vi "Read Sudoku String.vi"(8 "error in (no error)":errorcluster, 11 "Sudoku Class in":refnum<class "Sudoku Class.lvclass">) -> (0 "error out":errorcluster, 2 "Sudoku String":T1, 3 "Sudoku Class out":refnum<class "Sudoku Class.lvclass">)   [LabVIEW 2015, in "Sudoku Library.lvlib" / "Sudoku Class.lvclass"]
doc: "Created IvanLis by LabVIEW Portal\nProfile: http://labviewportal.org/memberlist.php?mode=viewprofile&u=987\neMail: IvanLisanov@gMail.com\nTelegram: https://t.me/IvanLis"
uses:
  Sudoku Class.lvclass
  TypeDef/Sudoku String.ctl
  Sudoku Class.lvclass/Sudoku Class.ctl
  Sudoku Library.lvlib
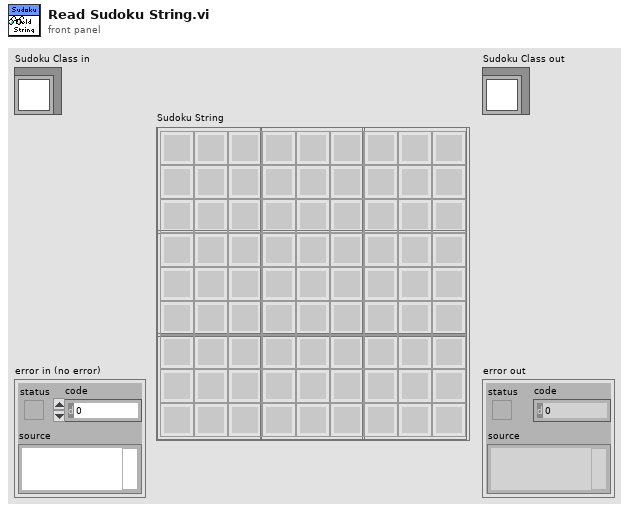
[diagram p1: front panel]
types:
  T1 = typedef "Sudoku Library.lvlib/Sudoku String.ctl" = string[][]
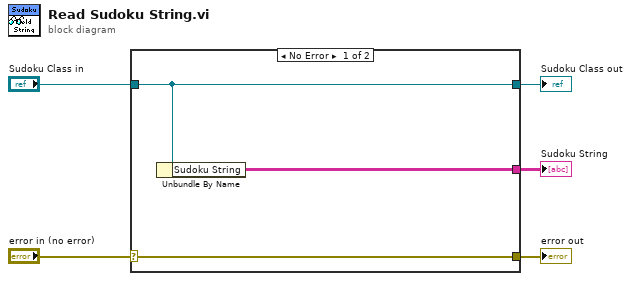
[diagram p0: block diagram]
diagram:
  n1 = case shown="No Error" "error in (no error)" {
    selector: "error in (no error)" -> [w8 w9]
    tunnel: [w8 w9] -> w4
    tunnel: [w7 w10] -> w2
    tunnel: "Sudoku Class in" -> [w7 w10]
    tunnel: [w6 _] -> w1
    frame No Error {
      n2 = Unbundle By Name(w7) -> ("Sudoku String"=w6:T1)
    }
    frame Error {
    }
  }
  "error out" <- w4
  "Sudoku Class out" <- w2
  "Sudoku String" <- w1
